vi "Analogico_digital.vi"(0 "Array":sgl[](array[numeric]), 1 "Offset WS":sgl, 3 "Frecuencia muestreo":dbl) -> (7 "array w/ subset deleted":sgl[](array[numeric]), 10 "Tiempo\npaso":dbl)   [LabVIEW 2015]
panel:
  out "Primer punto":i32
  out "Último punto":i32
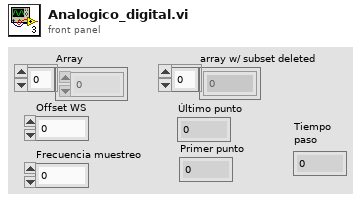
[diagram p1: front panel]
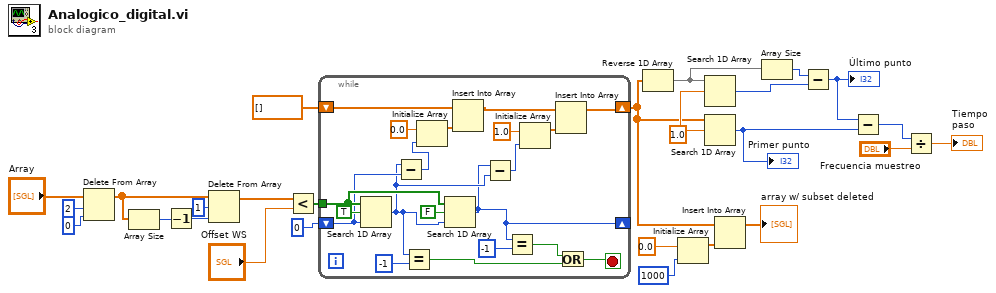
[diagram p0: block diagram]
diagram:
  w10 = sgl 1.0 ("element")
  n1 = Delete From Array(array="Array", length=2, index=0) -> (array with subset deleted=w18:sgl[])  [unwired: 1 out]
  n2 = Array Size(array=w18) -> (size(s)=w16:i32)
  n3 = Decrement(x=w16) -> (x-1=w17:i32)
  n4 = Delete From Array(array=w18, length=1, index=w17) -> (array with subset deleted=w13:sgl[])  [unwired: 1 out]
  n5 = Less?(x=w13, y="Offset WS") -> (x < y?=w21:bool[])
  n6 = while {
    shift-right: [w34] -> w9
    shift-left: sgl[] [] ("array w/ subset deleted") -> [w43]
    tunnel: w21 -> [w44]
    shift-right: [w29] -> _
    shift-left: 0 ("index") -> [w37]
    stop <- w30 stop-if-true
    n7 = Search 1D Array(1D array=w44, element=TRUE, start index (0)=w37) -> (index of element=w33:i32)
    n8 = Subtract(x=w33, y=w37) -> (x-y=w36:i32)
    n9 = Equal?(x=w33, y=-1) -> (x = y?=w27:bool)
    n10 = Initialize Array(0.0 ("element"), w36) -> (w41:dbl[])
    n11 = Search 1D Array(1D array=w44, element=FALSE, start index (0)=w33) -> (index of element=w29:i32)
    n12 = Insert Into Array(array=w43, new element=w41) -> (w38:sgl[])  [unwired: 1 in]
    n13 = Subtract(x=w29, y=w33) -> (x-y=w35:i32)
    n14 = Equal?(x=w29, y=-1) -> (x = y?=w28:bool)
    n15 = Initialize Array(1.0 ("element"), w35) -> (w39:dbl[])
    n16 = Insert Into Array(array=w38, new element=w39) -> (w34:sgl[])  [unwired: 1 in]
    n17 = Or(x=w28, y=w27) -> (x .or. y?=w30:bool)
  }
  n18 = Reverse 1D Array(array=w9) -> (reversed array=w8:sgl[])
  n19 = Initialize Array(0.0 ("element"), 1000 ("dimension size")) -> (w24:dbl[])
  n20 = Search 1D Array(1D array=w8, element=w10) -> (index of element=w6:i32)  [unwired: 1 in]
  n21 = Search 1D Array(1D array=w9, element=w10) -> (index of element=w4:i32)  [unwired: 1 in]
  "Primer punto" <- w4
  n22 = Insert Into Array(array=w9, new element=w24) -> (→"array w/ subset deleted":sgl[])  [unwired: 1 in]
  n23 = Array Size(array=w8) -> (size(s)=w7:i32)
  n24 = Subtract(x=w7, y=w6) -> (x-y=w5:i32)
  "Último punto" <- w5
  n25 = Subtract(x=w5, y=w4) -> (x-y=w2:i32)
  n26 = Divide(x=w2, y="Frecuencia muestreo") -> (x/y=→"Tiempo\npaso":dbl)
